vi "Dashboard Main.vi"() -> ()   [LabVIEW 2016]
uses:
  <vilib>/Utility/miscctls.llb/LVRowAndColumnTypeDef.ctl
  <vilib>/event_ctls.llb/eventvkey.ctl
  <vilib>/Rock Robotics/Network Tables/NT Read Numeric Array.vi
  <vilib>/Rock Robotics/Network Tables/NT Read Boolean.vi
  <vilib>/Rock Robotics/WPI/Dashboard/WPI_DashboardLogging Global.vi
panel:
  in  "Camera Settings Right":T1={"Frame Rate"=30, "Compression"=30, "Size"=1, "DB Camera Config"=FALSE} {"Frame Rate" scale=1.0..30.0; "Compression" scale=100.0..-1.0; "Size" items=["640x480", "320x240", "160x120"]}
  in  "Camera Name Right":string(combo)="No Camera Selection"
  out "Camera Info":cluster{"Mbps LED":bool, "Mbps":dbl, "fps":dbl} {"fps" format="%#.1g"; "Mbps" format="%#.1g"}
  in  "Camera Settings":T1={"Frame Rate"=30, "Compression"=30, "Size"=1, "DB Camera Config"=FALSE} {"Frame Rate" scale=1.0..30.0; "Compression" scale=100.0..-1.0; "Size" items=["640x480", "320x240", "160x120"]}
  in  "TCP":refnum<k5>
  in  "Rec Mode":enum32{"Stop", "Record", "Playback"}(radio)
  out "Robot IP":string
  out "Image Message":string="Timeout in Camera Communications"
  in  "Dashboard Tab":T2(tab)
  out "Waveform Chart":dbl[][](graph)
  out "Good to Shoot?":bool
  out "NT Connection":bool
  out "MotorChart R":cluster{"Numeric":dbl, "Numeric":dbl}(graph)
  out "MotorChart L":cluster{"Numeric":dbl, "Numeric":dbl}(graph)
  out "MotorSliders R":cluster{"MotorSlide1":dbl, "MotorSlide2":dbl} {"MotorSlide2" scale=-1.0..1.0 scale format="%#_2e"; "MotorSlide1" scale=-1.0..1.0 scale format="%#_2e"}
  out "MotorSliders L":cluster{"MotorSlide1":dbl, "MotorSlide2":dbl} {"MotorSlide2" scale=-1.0..1.0 scale format="%#_2e"; "MotorSlide1" scale=-1.0..1.0 scale format="%#_2e"}
  out "Gyro":dbl(knob) scale=0.0..360.0
  out "JS1 Z":dbl(slide) scale=-1.0..1.0 scale format="%#_2e"
  out "JS1 Graph":cluster{"X":dbl, "Y":dbl}[](graph)
  out "JS1 Buttons":T3
  out "JS2 Z":dbl(slide) scale=-1.0..1.0 scale format="%#_2e"
  out "JS2 Graph":cluster{"X":dbl, "Y":dbl}[](graph)
  out "JS2 Buttons":T3
  out "Mode":T4(ring)=enum."Auto Disabled"
  in  "Auto List":string(combo)="Select Autonomous ..."
  out "Camera Image Right":T5(plugin-control)
  in  "DB/String 9":string
  in  "DB/String 8":string
  in  "DB/String 7":string
  in  "DB/String 6":string
  in  "DB/String 5":string
  in  "DB/String 4":string
  in  "DB/String 3":string
  in  "DB/String 2":string
  in  "DB/String 1":string
  in  "DB/String 0":string
  in  "DB/Slider 0":dbl(slide) scale=0.0..5.0
  in  "DB/Slider 1":dbl(slide) scale=0.0..5.0
  in  "DB/Slider 2":dbl(slide) scale=0.0..5.0
  in  "DB/Slider 3":dbl(slide) scale=0.0..5.0
  out "DB/LED 3":bool
  out "DB/LED 2":bool
  out "DB/LED 1":bool
  out "DB/LED 0":bool
  in  "DB/Button 3":bool
  in  "DB/Button 2":bool
  in  "DB/Button 1":bool
  in  "DB/Button 0":bool caption="New Name"
  in  "Test Slider":dbl(slide) scale=0.0..100.0 scale format="%#_3g"
  in  "On/Off":bool caption="Solenoid"
  in  "Test Name":u16(ring) items=["Select the test to run..."]
  in  "Test Tree":string(tree)
  in  "Motor":cluster{"Value":dbl, "Enable":bool} {"Value" scale=-1.0..1.0 scale format="%#_3g"}
  out "Progress":T6 {"Test Progress" scale=0.0..100.0}
  in  "Rev/Fwd":cluster{"Forward":bool, "Reverse":bool}
  in  "Test Ring":u16(ring) items=["Monochrome", "Color"]
  out "Cmd Status":string
  in  "Execute Command":bool
  in  "Command Params":string[][](table)
  in  "Command Selection":i32(listbox)
  in  "CheckList":i32(listbox)
  out "Tree":string(tree)
  out "Camera Image":T5(plugin-control)
  out "Background":bool
  in  "Camera Name":string(combo)="No Camera Selection"
  # "HW"
  # "HW"
  # "Joysticks"
  # "Drive Motors"
  # "Front"
  # "Right"
  # "Left"
  # "Back"
  # "This tab is a great place for autonomous settings and robot-specific values.\nPlace controls and indicators inside this tab and match name to\nDashboard Variables on robot. You can also delete this comment."
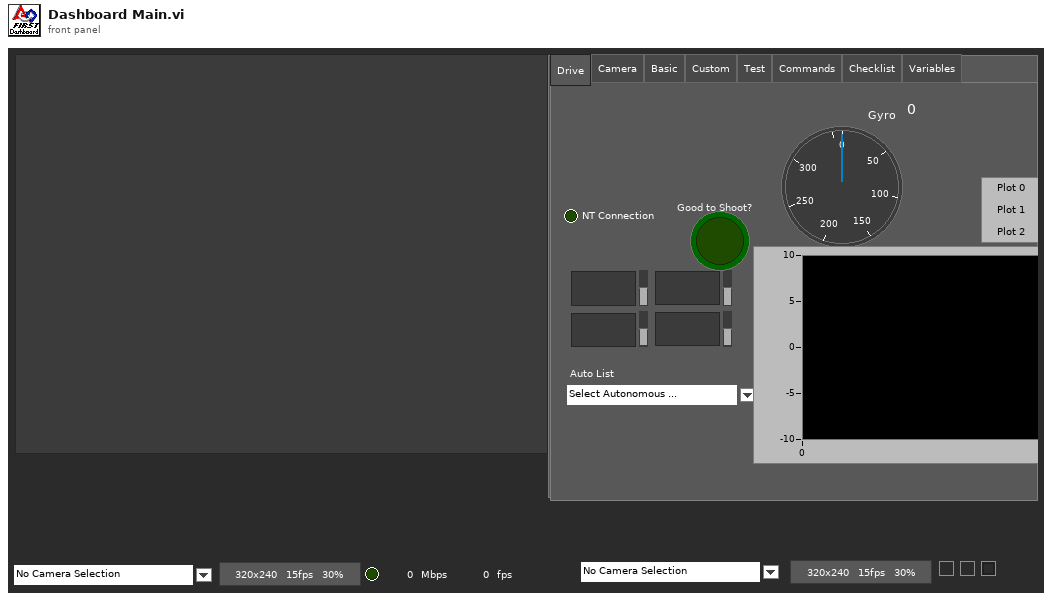
[diagram p1: front panel]
types:
  T1 = cluster{"Frame Rate":i32, "Compression":i32, "Size":u16, "DB Camera Config":bool}
  T2 = enum32{"Drive", "Camera", "Basic", "Custom", "Test", "Commands", "Checklist", "Variables"}
  T3 = cluster{bool, bool, bool, bool, bool, bool, bool, bool, bool, bool, bool, bool}
  T4 = enum8{"Tele-Op Disabled", "Tele-Op Enabled", "Auto Disabled", "Auto Enabled", "Test Disabled", "Test Enabled", "Disconnected", "No Code", "E-Stop"}
  T5 = typedef "IMAQ Image.ctl" = refnum<image>
  T6 = cluster{"Test Progress":u8, "Test Progress Text":string}
  T7 = typedef "Image Type" = u32
  T8 = cluster{"IDs":cluster{"RPC field ID":u16, "Unique ID":u16}, "String":string}
  T9 = enum32{"Drive", "Basic", "Custom", "Test", "Checklist", "Variables"}
  T10 = cluster{"Error Strings":string, "Disable Counts":cluster{u16, u16}, "Rail Faults":cluster{u16, u16, u16}, "Robot IP":string, "DB Mode":u8, "Event Info":cluster{"Name":string, "Type":u8, "Number":u16, "Replay":u8}}
  T11 = cluster{"Storage":cluster{"Disk Free":u64, "RAM Block":u32, "RAM free":u32}, "CPU Utilization":cluster{"CPU % ISR":sgl, "CPU % Time Crit":sgl, "CPU % Timed Str":sgl, "CPU % High":sgl, "CPU % Above":sgl, "CPU % Normal":sgl, "CPU % Low":sgl}, "CAN":cluster{"% Bus Utilization":sgl, "Bus Off Cnt":u32, "TX_FIFO Full Cnt":u32, "Receive Error Cnt":u8, "Transmit Error Cnt":u8}, "HID":cluster{"HID Outputs":u32, "Rumble Low":u16, "Rumble High":u16}[]}
  T12 = cluster{"Status bits":cluster{"Test Mode":bool, "Autonomous":bool, "Enabled":bool, "Code Start":bool, "Brownout":bool, "Reserved 2":bool, "Reserved 3":bool, "E-Stop":bool}, "Code Trace":cluster{"Disabled":bool, "TeleOp":bool, "Auto":bool, "Test":bool}, "Controller Type":enum16{"unknown", "cRIO", "roboRio"}, "Code?":enum16{"unknown", "noCode", "code"}, "Battery V":dbl}
  T13 = cluster{"Control Bits":cluster{"TestMode":bool, "Autonomous":bool, "Enabled":bool, "FMS Present":bool, bool, bool, bool, "E-Stop":bool}, "Team Station ":u8, "Countdown":sgl, "Joystick Values":cluster{"Axes":dbl[], "Buttons":bool[], "POVs":i16[]}[]}
  T14 = cluster{"Axes":dbl[], "Buttons":bool[], "POVs":i16[]}[]
  T15 = cluster{"Axes":dbl[], "Buttons":bool[], "POVs":i16[]}
  T16 = cluster{"Buttons[0]":bool, "Buttons[1]":bool, "Buttons[2]":bool, "Buttons[3]":bool, "Buttons[4]":bool, "Buttons[5]":bool, "Buttons[6]":bool, "Buttons[7]":bool, "Buttons[8]":bool, "Buttons[9]":bool, "Buttons[10]":bool, "Buttons[11]":bool}
  T17 = cluster{"Camera Image":refnum<vi>, "Dashboard Tab":refnum<vi>, "Background":refnum<vi>, "Rec Mode":refnum<vi>, "Test Slider":refnum<vi>, "On/Off ":refnum<vi>, "Test Ring":refnum<vi>, "Rev/Fwd":refnum<vi>, "Test Name":refnum<vi>, "Motor":refnum<vi>, "Progress":refnum<vi>, "CheckList":refnum<vi>, "Tree":refnum<vi>, "Test Tree":refnum<vi>, "Command Params":refnum<vi>, "Command Selection":refnum<vi>, "Execute Command":refnum<vi>, "Cmd Status":refnum<vi>, "Camera Settings":refnum<vi>, "Camera Name":refnum<vi>, "Camera Info":refnum<vi>, "Camera Settings Right":refnum<vi>, "Camera Name Right":refnum<vi>, "Camera Image Right":refnum<vi>}
  T18 = cluster{"Operation":enum16{"Update", "Clear"}, "Color Box":u32}[]
  T19 = typedef "eventvkey.ctl" = enum16{"ASCII", "Enter", "Return", "Shift", "Ctrl", "Alt", "Cmd", "Opt", "Caps", "NumLock", "Clear", "Break", "Up", "Down", "Left", "Right", "Insert", "Delete", "Home", "End", "PageUp", "PageDown", "Escape", "Help", "Pause", "ScrollLock", "F1", "F2", "F3", "F4", "F5", "F6", "F7", "F8", "F9", "F10", "F11", "F12", "F13", "F14", "F15", "F16", "F17", "F18", "F19", "F20", "F21", "F22", "F23", "F24", "Play", "VolumeUp", "VolumeDown", "Mute", "Two Byte Char"}
  T20 = cluster{"Image Size":bool, "Image Type":bool, "Pixel Value":bool, "ROI Information":bool, "Zoom Factor":bool}
  T21 = cluster{"Operation":enum16{"Update", "Clear"}, "Color Box":u32}
  T22 = typedef "LVRowAndColumnTypeDef.ctl" = cluster{"Row":i32, "Column":i32}
  T23 = cluster{"Shift":bool, "Ctrl":bool, "Alt":bool, "Cmd":bool, "Opt":bool}
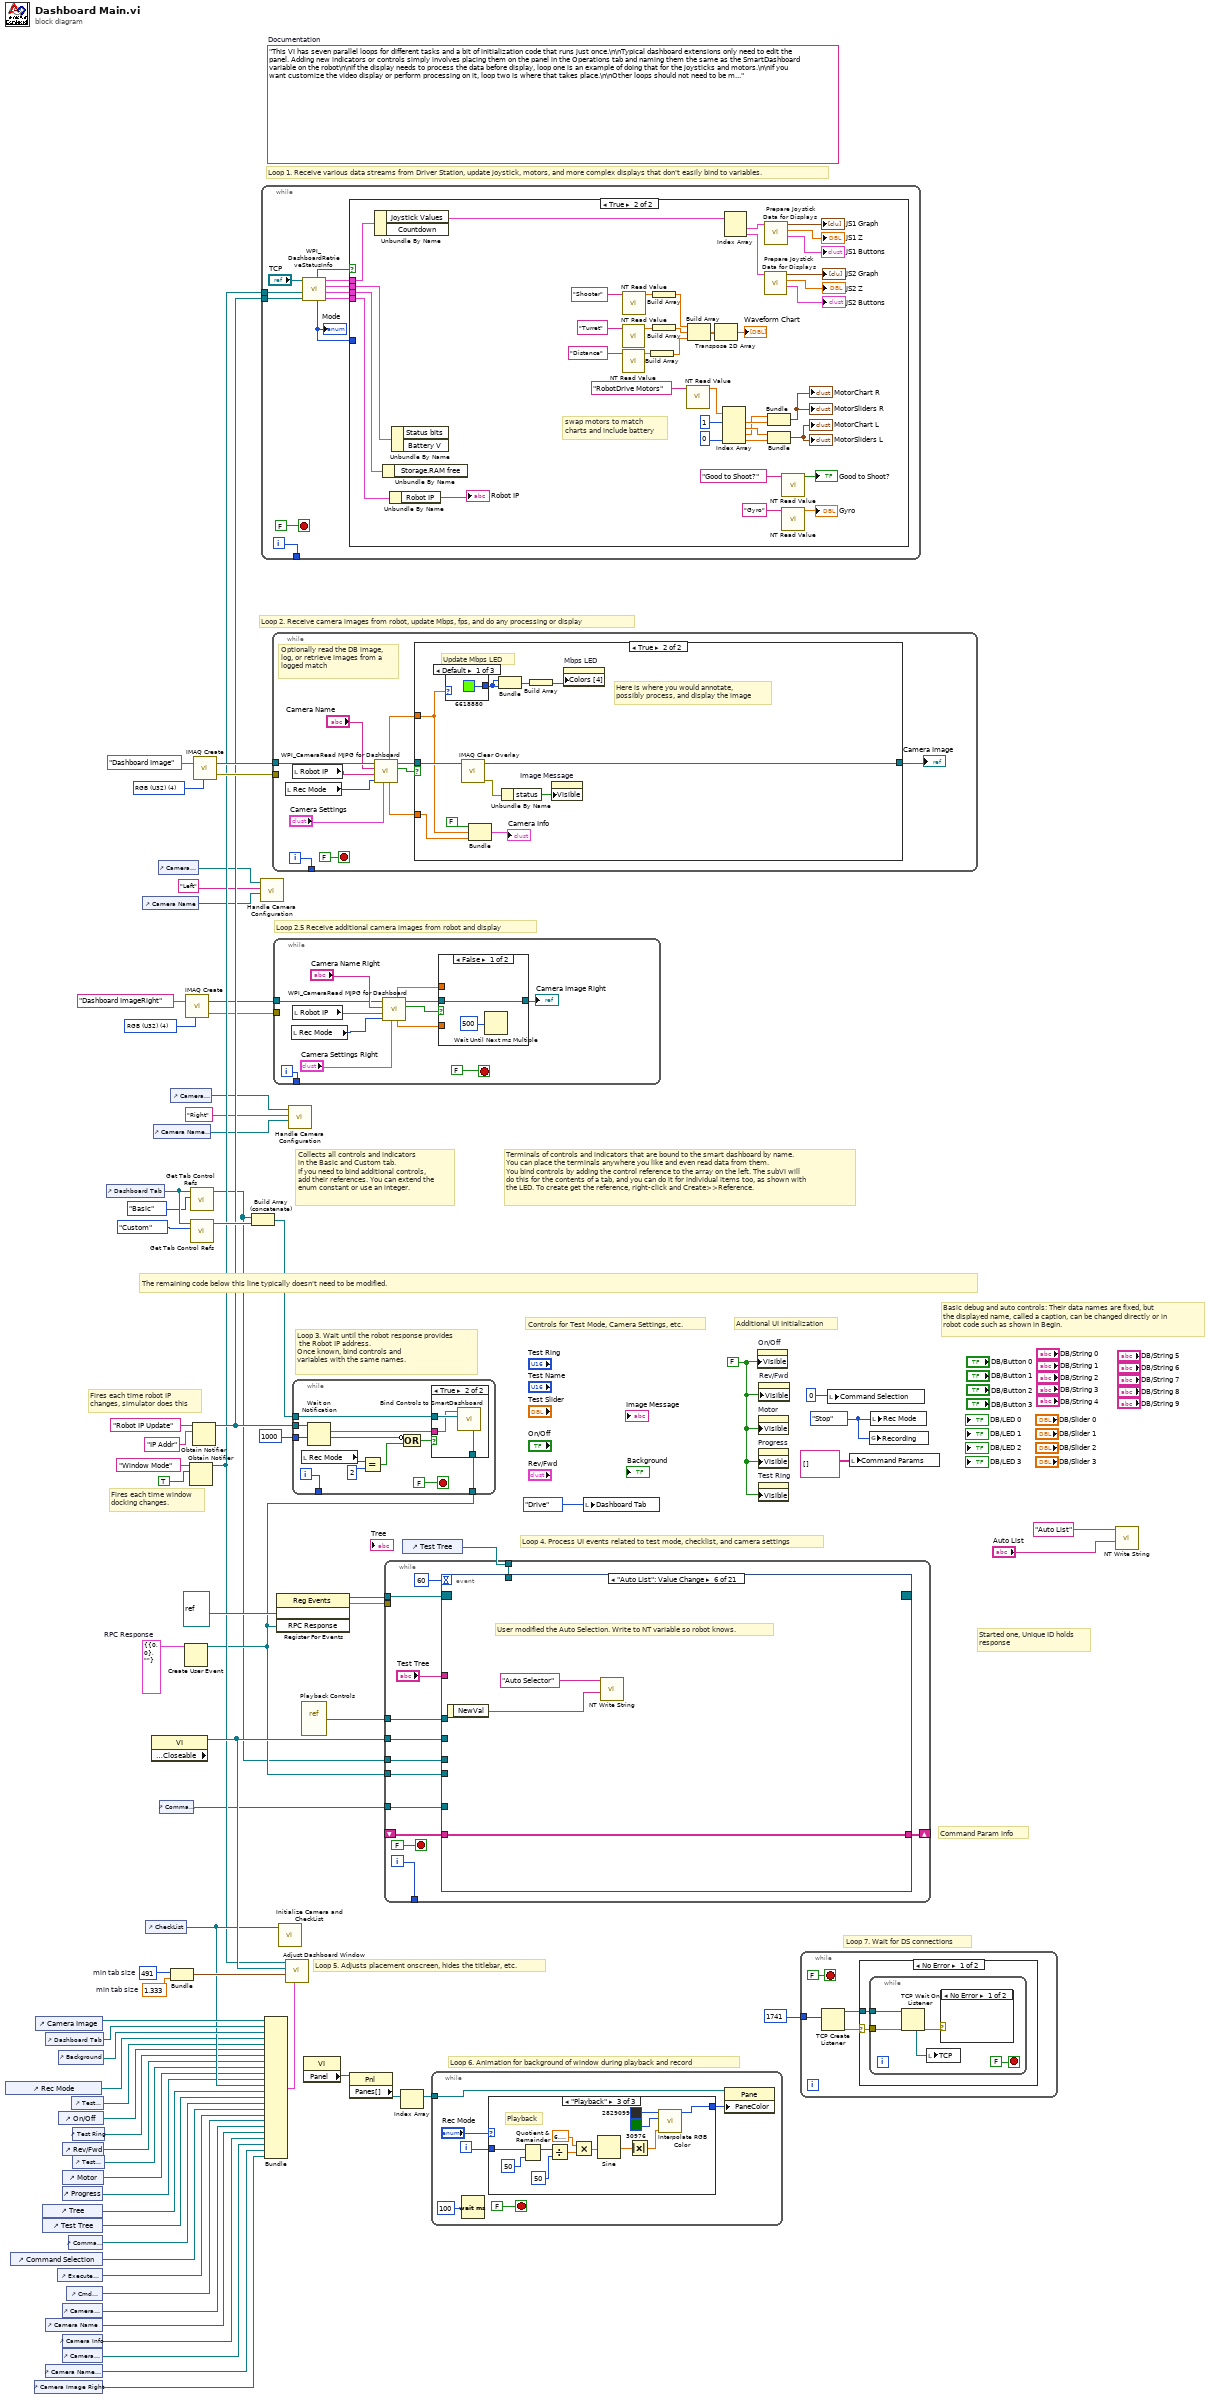
[diagram p0: block diagram]
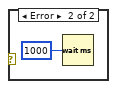
[diagram p3: hidden frame]
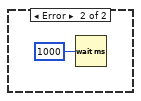
[diagram p4: hidden frame]
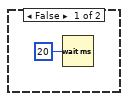
[diagram p5: hidden frame]
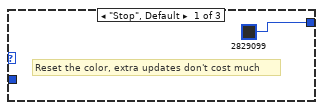
[diagram p6: hidden frame]
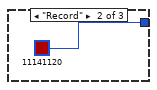
[diagram p7: hidden frame]
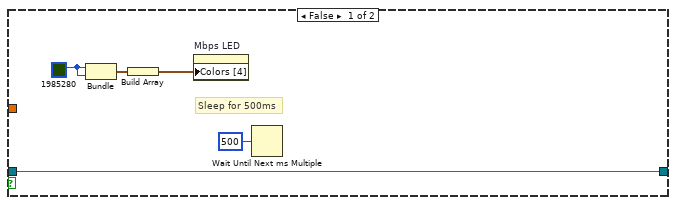
[diagram p9: hidden frame]
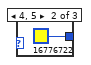
[diagram p10: hidden frame]
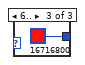
[diagram p11: hidden frame]
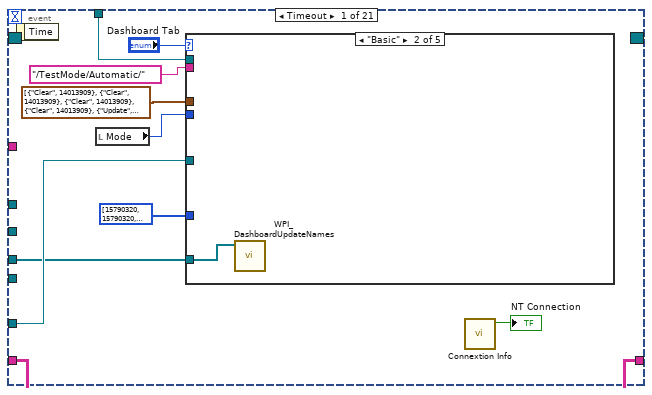
[diagram p12: hidden frame]
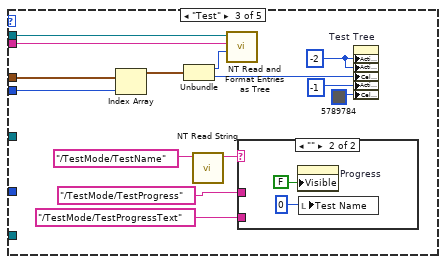
[diagram p14: hidden frame]
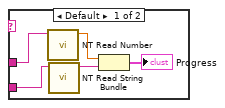
[diagram p15: hidden frame]
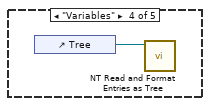
[diagram p16: hidden frame]
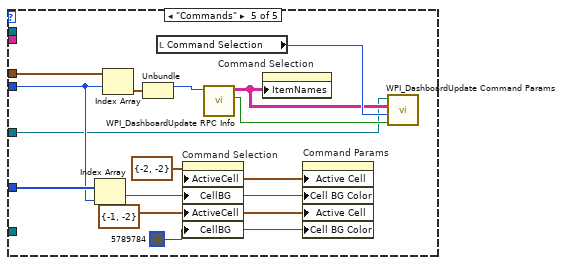
[diagram p17: hidden frame]
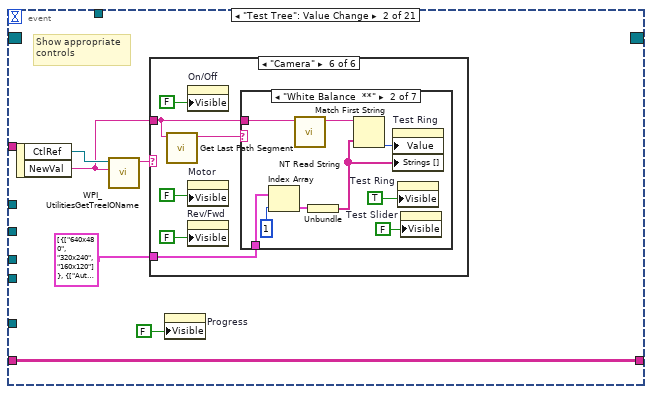
[diagram p18: hidden frame]
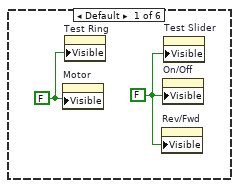
[diagram p19: hidden frame]
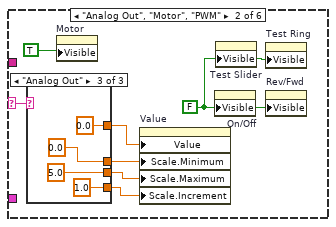
[diagram p20: hidden frame]
diagram:
  w12 = T7 4 items=["Grayscale (U8)", "Grayscale (I16)", "Grayscale (SGL)", "Complex (CSG)", "RGB (U32)", "HSL (U32)", "RGB (U64)"] ("Image Type")
  w26 = T8 {"IDs"={"RPC field ID"=0, "Unique ID"=0}, "String"=""}  # RPC Response
  w51 = 491  # min tab size
  w50 = 1.333  # min tab size
  w58 = enum32{"Stop", "Record", "Playback"}."Stop" ("Rec Mode")
  w33 = FALSE ("Visible")
  (unwired) "This VI has seven parallel loops for different tasks and a bit of initialization code that runs just once.\n\nTypical dashboard extensions only need to edit the panel. Adding new indicators or controls simply involves placing them on the panel in the Operations tab and naming them the same as the SmartDashboard variable on the robot\n\nIf the display needs to process the data before display, loop one is an example of doing that for the joysticks and motors.\n\nIf you want customize the video display or perform processing on it, loop two is where that takes place.\n\nOther loops should not need to be modified. They are pretty standard, and document the task they perform."  # Documentation
  w75 = T7 4 items=["Grayscale (U8)", "Grayscale (I16)", "Grayscale (SGL)", "Complex (CSG)", "RGB (U32)", "HSL (U32)", "RGB (U64)"] ("Image Type")
  # "Loop 2.5 Receive additional camera images from robot and display"
  # "Command Param Info"
  # "Started one, Unique ID holds\nresponse"
  # "Loop 7. Wait for DS connections"
  # "Basic debug and auto controls: Their data names are fixed, but\nthe displayed name, called a caption, can be changed directly or in\nrobot code such as shown in Begin."
  # "Controls for Test Mode, Camera Settings, etc."
  # "Additional UI Initialization"
  # "Loop 6. Animation for background of window during playback and record"
  # "Fires each time robot IP\nchanges, simulator does this"
  # "Fires each time window\ndocking changes."
  # "Collects all controls and indicators\nin the Basic and Custom tab.\nIf you need to bind additional controls,\nadd their references. You can extend the\nenum constant or use an integer."
  # "The remaining code below this line typically doesn't need to be modified."
  # "Loop 4. Process UI events related to test mode, checklist, and camera settings"
  # "Terminals of controls and indicators that are bound to the smart dashboard by name.\nYou can place the terminals anywhere you like and even read data from them.\nYou bind controls by adding the control reference to the array on the left. The subVI will\ndo this for the contents of a tab, and you can do it for individual items too, as shown with\nthe LED. To create get the reference, right-click and Create>>Reference."
  # "Loop 3. Wait until the robot response provides\n the Robot IP address.\nOnce known, bind controls and\nvariables with the same names."
  # "Loop 5. Adjusts placement onscreen, hides the titlebar, etc."
  # "Loop 1. Receive various data streams from Driver Station, update joystick, motors, and more complex displays that don't easily bind to variables."
  # "Loop 2. Receive camera images from robot, update Mbps, fps, and do any processing or display"
  n1 = control-ref of="Rec Mode"() -> (w39:refnum<vi>)
  n2 = control-ref of="Command Selection"() -> (w25:refnum<vi>)
  n3 = control-ref of="Camera Image Right"() -> (w3:refnum<vi>)
  n4 = control-ref of="Camera Image"() -> (w53:refnum<vi>)
  n5 = control-ref of="Tree"() -> (w43:refnum<vi>)
  n6 = control-ref of="Test Tree"() -> (w42:refnum<vi>)
  n7 = control-ref of="Dashboard Tab"() -> (w52:refnum<vi>)
  n8 = control-ref of="Camera Name"() -> (w16:refnum<vi>)
  n9 = control-ref of="Camera Name Right"() -> (w4:refnum<vi>)
  n10 = control-ref of="Execute Command"() -> (w27:refnum<vi>)
  n11 = control-ref of="Background"() -> (w48:refnum<vi>)
  n12 = control-ref of="On/Off"() -> (w37:refnum<vi>)
  n13 = control-ref of="Progress"() -> (w34:refnum<vi>)
  n14 = control-ref of="Camera Settings"() -> (w17:refnum<vi>)
  n15 = control-ref of="Camera Info"() -> (w15:refnum<vi>)
  n16 = control-ref of="Camera Settings Right"() -> (w5:refnum<vi>)
  n17 = control-ref of="Rev/Fwd"() -> (w35:refnum<vi>)
  n18 = control-ref of="Motor"() -> (w40:refnum<vi>)
  n19 = control-ref of="Cmd Status"() -> (w21:refnum<vi>)
  n20 = control-ref of="Command Params"() -> (w28:refnum<vi>)
  n21 = control-ref of="Test Slider"() -> (w38:refnum<vi>)
  n22 = control-ref of="Test Ring"() -> (w36:refnum<vi>)
  n23 = control-ref of="Test Name"() -> (w41:refnum<vi>)
  n24 = control-ref of="Dashboard Tab"() -> (w56:refnum<vi>)
  n25 = control-ref of="Camera Name"() -> (w18:refnum<vi>)
  n26 = control-ref of="CheckList"() -> (w44:refnum<vi>)
  n27 = property class="VI" props=["Front Panel.Closeable"]() -> (reference out=w57:refnum<vi>)  [unwired: 2 in, 2 out]
  n28 = control-ref of="Camera Name Right"() -> (w8:refnum<vi>)
  n29 = control-ref of="Camera Settings"() -> (w19:refnum<vi>)
  n30 = control-ref of="Command Params"() -> (w20:refnum<vi>)
  n31 = control-ref of="Camera Settings Right"() -> (w9:refnum<vi>)
  n32 = Bundle("min tab size"=w51, "min tab size"=w50) -> (w49:cluster{"min tab size":i32, "min tab size":dbl})  [unwired: 1 in]
  n33 = Create User Event(user event datatype=w26) -> (user event=w22:refnum<user-event>)  [unwired: 1 in, 1 out]
  n34 = call "IMAQ Create"("Image Name"="Dashboard ImageRight", "Image Type"=w12) -> ("New Image"=w11:T5, "error out"=w10:errorcluster)  [unwired: 2 in, 1 out]
  n35 = Obtain Notifier(name (unnamed)="Window Mode", notification data type=TRUE) -> (notifier out=w31:refnum<notifier>)  [unwired: 2 in, 2 out]
  n36 = call <vilib>:"Get Tab Control Refs.vi"("Page Index"=T9."Basic" ("Dashboard Tab"), "TabControl in"=w56) -> ("ControlsOnPage"=w14:refnum<vi>[])  [unwired: 9 in]
  n37 = call <vilib>:"Get Tab Control Refs.vi"("Page Index"=T9."Custom" ("Dashboard Tab"), "TabControl in"=w56) -> ("ControlsOnPage"=w55:refnum<vi>[])  [unwired: 9 in]
  n38 = Obtain Notifier(name (unnamed)="Robot IP Update", notification data type="IP Addr" ("name (unnamed)")) -> (notifier out=w32:refnum<notifier>)  [unwired: 2 in, 2 out]
  n39 = call "IMAQ Create"("Image Name"="Dashboard Image", "Image Type"=w75) -> ("New Image"=w73:T5, "error out"=w72:errorcluster)  [unwired: 2 in, 1 out]
  n40 = Build Array (concatenate)(w14, w55) -> (w54:refnum<vi>[])
  n41 = call "Handle Camera Configuration.vi"("CameraNameRef"=w18, "Camera File Name"="Left", "ClusterRef"=w19) -> ()  [unwired: 9 in]
  n42 = while {
    tunnel: [w85] -> _
    tunnel: w32 -> [w79]
    tunnel: w31 -> [w76]
    i -> [w85]
    stop <- FALSE stop-if-true
    n43 = call <vilib>:"WPI_DashboardRetrieveStatusInfo.vi"("Binding Refnum"=w79, "Window Mode Notifier"=w76, "TCP Cnx"="TCP") -> ("Power and Errors"=w80:T10, "Robot Metrics"=w83:T11, "Status Info"=w84:T12, "Control Info"=w81:T13, "Robot Mode"=w78:T4, "Process?"=w82:bool)  [unwired: 3 in]
    "Mode" <- w78
    n44 = case shown="True" w82 {
      tunnel: w84 -> [_ w126]
      tunnel: w83 -> [_ w125]
      tunnel: w81 -> [_ w124]
      tunnel: w80 -> [_ w123]
      tunnel: w78 -> [_ _]
      frame False {
        n45 = Wait (ms)(milliseconds to wait=u32 20) -> ()  [unwired: 1 out]
      }
      frame True {
        # "swap motors to match\ncharts and include battery"
        n46 = Unbundle By Name(w124) -> ("Joystick Values"=w114:T14)  [unwired: 1 out]
        n47 = Unbundle By Name(w125) -> ()  [unwired: 1 out]
        n48 = Unbundle By Name(w123) -> ("Robot IP"=→"Robot IP":string)
        n49 = Unbundle By Name(w126) -> ()  [unwired: 2 out]
        n50 = call-poly <vilib>:"NT Read Value.vi"("Name"="Turret") -> ("Numeric"=w94:dbl)  [unwired: 9 in, 1 out]
        n51 = call-poly <vilib>:"NT Read Value.vi"("Name"="Distance") -> ("Numeric"=w93:dbl)  [unwired: 9 in, 1 out]
        n52 = call-poly <vilib>:"NT Read Value.vi"("Name"="Shooter") -> ("Numeric"=w95:dbl)  [unwired: 9 in, 1 out]
        n53 = Build Array(w93) -> (w90:dbl[])
        n54 = Build Array(w95) -> (w92:dbl[])
        n55 = Build Array(w94) -> (w91:dbl[])
        n56 = call-poly <vilib>:"NT Read Value.vi"("Name"="RobotDrive Motors") -> ("Numeric Array"=w104:dbl[])  [unwired: 9 in, 1 out]
        n57 = Build Array(w92, w91, w90) -> (w89:dbl[][])
        n58 = Transpose 2D Array(2D array=w89) -> (transposed array=→"Waveform Chart":dbl[][])
        n59 = Index Array(array=w104, index #1=1, index #4=0) -> (element #1=w118:dbl, element #2=w119:dbl, element #3=w117:dbl, element #4=w122:dbl)  [unwired: 2 in]
        n60 = Index Array(array=w114) -> (element #1=w113:T15, element #2=w109:T15)  [unwired: 2 in]
        n61 = call "Prepare Joystick Data for Displays.vi"("Joystick Values"=w109) -> ("Buttons"=→"JS2 Buttons":T16, "Z Axis"=→"JS2 Z":dbl, "Cartesian Data"=→"JS2 Graph":cluster{"X axis":dbl, "X axis":dbl}[])  [unwired: 8 in]
        n62 = call "Prepare Joystick Data for Displays.vi"("Joystick Values"=w113) -> ("Buttons"=→"JS1 Buttons":T16, "Z Axis"=→"JS1 Z":dbl, "Cartesian Data"=→"JS1 Graph":cluster{"X axis":dbl, "X axis":dbl}[])  [unwired: 8 in]
        n63 = Bundle("Numeric"=w117, "Numeric"=w118) -> (→"MotorChart R" →"MotorSliders R":cluster{"Numeric":dbl, "Numeric":dbl})  [unwired: 1 in]
        n64 = Bundle("Numeric"=w119, "Numeric"=w122) -> (→"MotorChart L" →"MotorSliders L":cluster{"Numeric":dbl, "Numeric":dbl})  [unwired: 1 in]
        n65 = call-poly <vilib>:"NT Read Value.vi"("Name"="Good to Shoot?") -> ("Boolean"=→"Good to Shoot?":bool)  [unwired: 9 in, 1 out]
        n66 = call-poly <vilib>:"NT Read Value.vi"("Name"="Gyro") -> ("Numeric"=→"Gyro":dbl)  [unwired: 9 in, 1 out]
      }
    }
  }
  n67 = Bundle("Camera Image"=w53, "Dashboard Tab"=w52, "Background"=w48, "Rec Mode"=w39, "Test Slider"=w38, "On/Off"=w37, "Test Ring"=w36, "Rev/Fwd"=w35, "Test Name"=w41, "Motor"=w40, "Progress"=w34, "CheckList"=w44, "Tree"=w43, "Test Tree"=w42, "Command Params"=w28, "Command Selection"=w25, "Execute Command"=w27, "Cmd Status"=w21, "Camera Settings"=w17, "Camera Name"=w16, "Camera Info"=w15, "Camera Settings Right"=w5, "Camera Name Right"=w4, "Camera Image Right"=w3) -> (w45:T17)  [unwired: 1 in]
  n68 = while {
    tunnel: w73 -> [w136]
    tunnel: w72 -> [_]
    tunnel: [w137] -> _
    i -> [w137]
    stop <- FALSE stop-if-true
    # "Optionally read the DB image,\nlog, or retrieve images from a\nlogged match"
    n69 = local read "Rec Mode"() -> (w132:enum32{"Stop", "Record", "Playback"})
    n70 = local read "Robot IP"() -> (w131:string)
    n71 = call <vilib>:"WPI_CameraRead MJPG for Dashboard.vi"("Camera Settings"="Camera Settings", "Rec Mode"=w132, "Robot IP"=w131, "Camera Name"="Camera Name", "Refnum in"=w136) -> ("Active"=w134:bool, "Refnum out"=w135:T5, "FPS"=w133:dbl, "Bandwidth (Mbps)"=w130:dbl)  [unwired: 3 in]
    n72 = case shown="True" w134 {
      tunnel: w135 -> [w139 w150]
      tunnel: w130 -> [_ w147]
      tunnel: w133 -> [_ w148]
      tunnel: [w139 w144] -> w127
      frame False {
        w141 = u32 1985280 ("Color Box")
        # "Sleep for 500ms"
        n73 = Bundle("Color Box"=w141, "Color Box"=w141) -> (w142:cluster{"Color Box":u32, "Color Box":u32})  [unwired: 1 out]
        n74 = Build Array(w142) -> (w140:cluster{"Color Box":u32, "Color Box":u32}[])
        n75 = property on="Mbps LED" class="Bool (strict)"("Colors [4]"=w140) -> ()  [unwired: 2 in, 2 out]
        n76 = Wait Until Next ms Multiple(millisecond multiple=u32 500) -> ()  [unwired: 1 out]
      }
      frame True {
        # "Here is where you would annotate,\npossibly process, and display the image"
        # "Update Mbps LED"
        n77 = case shown="Default" w147 {
          tunnel: [u32 6618880 ("Color Box") u32 16776722 ("Color Box") u32 16716800 ("Color Box")] -> w151
          frame Default {
          }
          frame 4, 5 {
          }
          frame 6.. {
          }
        }
        n78 = call "IMAQ Clear Overlay"("Image"=w150) -> ("error out"=w153:errorcluster, "Image Out"=w144:T5)  [unwired: 2 in, 7 out]
        n79 = Bundle(FALSE, "Bandwidth (Mbps)"=w147, "FPS"=w148) -> (→"Camera Info":cluster{bool, "Bandwidth (Mbps)":dbl, "FPS":dbl})  [unwired: 1 in]
        n80 = Bundle("Color Box"=w151, "Color Box"=w151) -> (w152:cluster{"Color Box":u32, "Color Box":u32})  [unwired: 1 out]
        n81 = Unbundle By Name(w153) -> ("status"=w154:bool)
        n82 = Build Array(w152) -> (w149:cluster{"Color Box":u32, "Color Box":u32}[])
        n83 = property on="Image Message" class="Str"("Visible"=w154) -> ()  [unwired: 2 in, 2 out]
        n84 = property on="Mbps LED" class="Bool (strict)"("Colors [4]"=w149) -> ()  [unwired: 2 in, 2 out]
      }
    }
    "Camera Image" <- w127
  }
  n85 = while {
    tunnel: w11 -> [w168]
    tunnel: w10 -> [_]
    tunnel: [w162] -> _
    i -> [w162]
    stop <- FALSE stop-if-true
    n86 = local read "Rec Mode"() -> (w166:enum32{"Stop", "Record", "Playback"})
    n87 = local read "Robot IP"() -> (w167:string)
    n88 = call <vilib>:"WPI_CameraRead MJPG for Dashboard.vi"("Camera Settings"="Camera Settings Right", "Rec Mode"=w166, "Robot IP"=w167, "Camera Name"="Camera Name Right", "Refnum in"=w168) -> ("Active"=w161:bool, "Refnum out"=w164:T5, "FPS"=w159:dbl, "Bandwidth (Mbps)"=w160:dbl)  [unwired: 3 in]
    n89 = case shown="False" w161 {
      tunnel: w164 -> [w170 w172]
      tunnel: w160 -> [_ _]
      tunnel: w159 -> [_ _]
      tunnel: [w170 w172] -> w158
      frame False {
        n90 = Wait Until Next ms Multiple(millisecond multiple=u32 500) -> ()  [unwired: 1 out]
      }
      frame True {
      }
    }
    "Camera Image Right" <- w158
  }
  n91 = register-events(refnum<vi> refnum, w22) -> (reference out=w62:refnum<event-registration>, error out=w61:errorcluster)  [unwired: 2 in]
  n92 = call "Initialize Camera and CheckList.vi"("ListBox in"=w44) -> ()  [unwired: 11 in]
  n93 = call "Adjust Dashboard Window.vi"("Sizing Refnums"=w45, "Size Constraints"=w49, "VI"=w57, "WIn Mode"=w31) -> ()  [unwired: 8 in]
  n94 = call "Handle Camera Configuration.vi"("CameraNameRef"=w8, "Camera File Name"="Right", "ClusterRef"=w9) -> ()  [unwired: 9 in]
  n95 = while {
    tunnel: w54 -> [w184]
    tunnel: w32 -> [w182]
    tunnel: [w180] -> _
    tunnel: u32 1000 ("milliseconds to wait") -> [w179]
    tunnel: w22 -> [w173]
    i -> [w180]
    stop <- FALSE stop-if-true
    n96 = local read "Rec Mode"() -> (w175:enum32{"Stop", "Record", "Playback"})
    n97 = Wait on Notification(notifier=w182, timeout in ms (-1)=w179) -> (notification=w181:string, timed out?=w177:bool)  [unwired: 2 in, 2 out]
    n98 = Equal?(x=w175, y=u16 2 ("Rec Mode")) -> (x = y?=w176:bool)
    n99 = Compound Arithmetic op=OR(invert w177, w176) -> (w178:bool)
    n100 = case shown="True" w178 {
      tunnel: w184 -> [_ w187]
      tunnel: w181 -> [_ w186]
      tunnel: w173 -> [_ w185]
      frame False {
      }
      frame True {
        n101 = call <vilib>:"Bind Controls to SmartDashboard.vi"("RPC ref"=w185, "Bound Control Refs"=w187, "Server IP Address"=w186) -> ()  [unwired: 9 in]
      }
    }
  }
  n102 = vi-ref "Playback Controls.vi"() -> (w63:refnum<vi>)
  n103 = property class="VI"() -> ("Panel"=w65:refnum<vi>)  [unwired: 2 in, 2 out]
  n104 = property class="Pnl"(reference=w65) -> ("Panes[]"=w66:refnum<vi>[])  [unwired: 1 in, 2 out]
  n105 = Index Array(array=w66) -> (element=w64:refnum<vi>)  [unwired: 1 in]
  n106 = control-ref of="Test Tree"() -> (w67:refnum<vi>)
  n107 = while {
    tunnel: [w197] -> _
    tunnel: w67 -> [w196]
    tunnel: w63 -> [w195]
    tunnel: w62 -> [w194]
    tunnel: w61 -> [_]
    tunnel: w57 -> [w193]
    tunnel: w22 -> [w192]
    tunnel: w20 -> [w191]
    shift-right: [w190] -> _
    shift-left: _ -> [w189]
    tunnel: w14 -> [w188]
    i -> [w197]
    stop <- FALSE stop-if-true
    n108 = event shown="[5] \"Auto List\": Value Change" {
      selector: w194 -> [_ _ _ _ _ _ _ _ _ _ _ _ _ _ _ _ _ _ _ _ _]
      dyn-events: [_ _ _ _ _ _ _ _ _ _ _ _ _ _ _ _ w453 _ _ _ _] -> _
      timeout: u32 60 ("milliseconds to wait") -> [_ _ _ _ _ _ _ _ _ _ _ _ _ _ _ _ _ _ _ _ _]
      tunnel: w196 -> [w209 _ _ _ _ _ _ _ _ _ _ _ _ _ _ _ _ _ _ _ _]
      tunnel: "Test Tree" -> [_ _ _ _ _ _ _ _ _ _ _ w420 w428 w430 w434 w442 _ _ _ _ _]
      tunnel: w195 -> [_ _ _ _ _ _ _ _ _ _ _ _ _ _ _ _ w455 _ w473 _ _]
      tunnel: w193 -> [_ _ _ _ _ _ _ _ _ _ _ _ _ _ _ _ w451 _ _ _ _]
      tunnel: w192 -> [_ _ _ _ _ _ _ _ _ _ _ _ _ _ _ _ w447 _ _ _ _]
      tunnel: w191 -> [w204 _ _ _ _ _ w371 _ _ _ _ _ _ _ _ _ _ _ _ _ _]
      tunnel: [w203 w248 w350 w355 w364 w368 w369 w378 w388 w395 w407 w419 w426 w429 w433 w441 w446 w468 w470 w474 w485] -> w190
      tunnel: w189 -> [w203 w248 w350 w355 w364 w368 w369 _ _ w395 w407 w419 w426 w429 w433 w441 w446 w468 w470 w474 w485]
      tunnel: w188 -> [w201 _ _ _ _ _ _ _ _ _ _ _ _ _ _ _ _ _ _ _ _]
      event Timeout {
        n109 = event-data() -> ()  [unwired: 1 in, 1 out]
        n110 = local read "Mode"() -> (w206:T4)
        n111 = case shown="\"Basic\"" "Dashboard Tab" {
          tunnel: w209 -> [_ _ w225 _ _]
          tunnel: "/TestMode/Automatic/" ("Name Pattern") -> [_ _ w224 _ _]
          tunnel: T18 [{"Operation"=enum."Clear", "Color Box"=14013909}, {"Operation"=enum."Clear", "Color Box"=14013909}, {"Operation"=enum."Clear", "Color Box"=14013909}, {"Operation"=enum."Clear", "Color Box"=14013909}, {"Operation"=enum."Update", "Color Box"=14013909}, {"Operation"=enum."Update", "Color Box"=16777215}, {"Operation"=enum."Clear", "Color Box"=14013909}, {"Operation"=enum."Clear", "Color Box"=14013909}, {"Operation"=enum."Clear", "Color Box"=14013909}] -> [_ _ w217 _ w241]
          tunnel: w206 -> [_ _ w216 _ w240]
          tunnel: u32[] [15790320, 15790320, 15790320, 15790320, 16777215, 16777215, 15790320, 15790320, 15790320] -> [_ _ _ _ w246]
          tunnel: w204 -> [_ _ _ _ w234]
          tunnel: w201 -> [_ w211 _ _ _]
          frame "Custom", Default {
          }
          frame "Basic" {
            n112 = call <vilib>:"WPI_DashboardUpdateNames.vi"("Controls on Tab"=w211) -> ()  [unwired: 11 in]
          }
          frame "Test" {
            w223 = -2 ("Active Item:Row Number")
            n113 = Index Array(array=w217, index=w216) -> (element=w218:T21)
            n114 = Unbundle(w218) -> ("Operation"=w219:enum16{"Update", "Clear"}, "Color Box"=w220:u32)
            n115 = call <vilib>:"NT Read String.vi"("Name"="/TestMode/TestName") -> ("String"=w214:string)  [unwired: 9 in, 1 out]
            n116 = call <vilib>:"NT Read and Format Entries as Tree.vi"("Operation"=w219, "Name Pattern"=w224, "Tree Refnum"=w225) -> ()  [unwired: 7 in, 2 out]
            n117 = case shown="\"\"" w214 {
              tunnel: "/TestMode/TestProgress" ("Name") -> [w227 _]
              tunnel: "/TestMode/TestProgressText" ("Name") -> [w226 _]
              frame Default {
                n118 = call <vilib>:"NT Read Number.vi"("Name"=w227) -> ("Numeric"=w228:dbl)  [unwired: 9 in, 1 out]
                n119 = call <vilib>:"NT Read String.vi"("Name"=w226) -> ("String"=w229:string)  [unwired: 9 in, 1 out]
                n120 = Bundle("Numeric"=w228, "String"=w229) -> (→"Progress":cluster{"Numeric":dbl, "String":string})  [unwired: 1 in]
              }
              frame "" {
                n121 = property on="Progress" class="Clust (strict)"("Visible"=FALSE) -> ()  [unwired: 2 in, 2 out]
                n122 = local write "Test Name"(u16 0) -> ()
              }
            }
            n123 = property on="Test Tree" class="Tree (strict)"("Active Item Row Number"=w223, "ActiveColNum"=w223, "CellBG"=w220, "Active Item Row Number"=-1 ("Active Item:Row Number"), "CellBG"=u32 5789784 ("Color Box")) -> ()  [unwired: 2 in, 2 out]
          }
          frame "Variables" {
            n124 = control-ref of="Tree"() -> (w233:refnum<vi>)
            n125 = call <vilib>:"NT Read and Format Entries as Tree.vi"("Tree Refnum"=w233) -> ()  [unwired: 9 in, 2 out]
          }
          frame "Commands" {
            w242 = u32 5789784 ("Color Box")
            w243 = T22 {"Row"=-1, "Column"=-2} ("Active Cell:Active Cell")
            w245 = T22 {"Row"=-2, "Column"=-2} ("Active Cell:Active Cell")
            n126 = Index Array(array=w246, index=w240) -> (element=w244:u32)
            n127 = Index Array(array=w241, index=w240) -> (element=w239:T21)
            n128 = Unbundle(w239) -> ("Operation"=w238:enum16{"Update", "Clear"})  [unwired: 1 out]
            n129 = local read "Command Selection"() -> (w237:i32)
            n130 = property on="Command Selection" class="MCListbox (strict)"("ActiveCell"=w245, "CellBG"=w244, "ActiveCell"=w243, "CellBG"=w242) -> ()  [unwired: 2 in, 2 out]
            n131 = call <vilib>:"WPI_DashboardUpdate RPC Info.vi"("Operation"=w238) -> ("update"=w236:bool, "commands"=w235:string[][])  [unwired: 9 in]
            n132 = property on="Command Selection" class="MCListbox (strict)"("ItemNames"=w235) -> ()  [unwired: 2 in, 2 out]
            n133 = property on="Command Params" class="Tbl (strict)"("Active Cell"=w245, "Cell BG Color"=w244, "Active Cell"=w243, "Cell BG Color"=w242) -> ()  [unwired: 2 in, 2 out]
            n134 = call <vilib>:"WPI_DashboardUpdate Command Params.vi"("Update"=w236, "NewVal"=w237, "Commands"=w235, "Param Tbl"=w234) -> ()  [unwired: 7 in, 1 out]
          }
        }
        n135 = call <vilib>:"Connextion Info.vi"() -> ("Connected"=→"NT Connection":bool)  [unwired: 10 in, 1 out]
      }
      event "Test Tree": Value Change {
        # "Show appropriate\ncontrols"
        n136 = event-data() -> ("CtlRef"=w251:refnum<vi>, "NewVal"=w249:string)  [unwired: 1 in]
        n137 = call <vilib>:"WPI_UtilitiesGetTreeIOName.vi"("NewVal"=w249, "TreeControl in"=w251) -> ("I/O Name"=w252:string)  [unwired: 9 in]
        n138 = case shown="\"Camera\"" w252 {
          selector: w252 -> [_ w259 _ w281 w290 _]
          tunnel: w249 -> [_ _ w278 w280 _ w297]
          tunnel: cluster{string[]}[] [{["640x480", "320x240", "160x120"]}, {["Auto", "Fixed indoor", "Fixed outdoor 1", "Fixed outdoor 2", "Fixed fluorescent 1", "Fixed fluorescent 2", "Hold current"]}, {["Auto", "Flicker-free 50 Hz", "Flicker-free 60 Hz", "Hold current"]}, {["None", "Prioritize frame rate", "Prioritize image quality"]}, {["Monochrome", "Color"]}] -> [_ _ _ _ _ w296]
          frame Default {
            w254 = FALSE ("Visible")
            w253 = FALSE ("Visible")
            n139 = property on="Motor" class="Clust (strict)"("Visible"=w253) -> ()  [unwired: 2 in, 2 out]
            n140 = property on="Test Ring" class="Ring (strict)"("Visible"=w253) -> ()  [unwired: 2 in, 2 out]
            n141 = property on="Rev/Fwd" class="Clust (strict)"("Visible"=w254) -> ()  [unwired: 2 in, 2 out]
            n142 = property on="On/Off" class="Bool (strict)"("Visible"=w254) -> ()  [unwired: 2 in, 2 out]
            n143 = property on="Test Slider" class="Slide (strict)"("Visible"=w254) -> ()  [unwired: 2 in, 2 out]
          }
          frame "Analog Out", "Motor", "PWM" {
            w260 = FALSE ("Visible")
            n144 = case shown="\"Analog Out\"" w259 {
              tunnel: [1.0 ("Value") -1.0 ("Value") 0.0 ("Value")] -> w258
              tunnel: [255.0 ("Value") 1.0 ("Value") 5.0 ("Value")] -> w257
              tunnel: [128.0 ("Value") 0.0 ("Value") 0.0 ("Value")] -> w256
              tunnel: [64.0 ("Value") 0.5 ("Value") 1.0 ("Value")] -> w255
              frame "PWM" {
              }
              frame "Motor", Default {
              }
              frame "Analog Out" {
              }
            }
            n145 = property on="Motor" class="Clust (strict)"("Visible"=TRUE) -> ()  [unwired: 2 in, 2 out]
            n146 = property on="Value" class="Slide (strict)"("Value"=w256, "Scale.Minimum"=w258, "Scale.Maximum"=w257, "Scale.Increment"=w255) -> ()  [unwired: 2 in, 2 out]
            n147 = property on="On/Off" class="Bool (strict)"("Visible"=w260) -> ()  [unwired: 2 in, 2 out]
            n148 = property on="Test Slider" class="Slide (strict)"("Visible"=w260) -> ()  [unwired: 2 in, 2 out]
            n149 = property on="Test Ring" class="Ring (strict)"("Visible"=w260) -> ()  [unwired: 2 in, 2 out]
            n150 = property on="Rev/Fwd" class="Clust (strict)"("Visible"=w260) -> ()  [unwired: 2 in, 2 out]
          }
          frame "Servo" {
            w276 = FALSE ("Visible")
            n151 = call <vilib>:"NT Read Number.vi"("Name"=w278) -> ("Numeric"=w277:dbl)  [unwired: 9 in, 1 out]
            n152 = property on="Test Slider" class="Slide (strict)"("Visible"=TRUE, "Scale.Maximum"=170.0 ("Scale.Range:Maximum")) -> ()  [unwired: 2 in, 2 out]
            n153 = local write "Test Slider"(w277) -> ()
            n154 = property on="Motor" class="Clust (strict)"("Visible"=w276) -> ()  [unwired: 2 in, 2 out]
            n155 = property on="Rev/Fwd" class="Clust (strict)"("Visible"=w276) -> ()  [unwired: 2 in, 2 out]
            n156 = property on="On/Off" class="Bool (strict)"("Visible"=w276) -> ()  [unwired: 2 in, 2 out]
            n157 = property on="Test Ring" class="Ring (strict)"("Visible"=w276) -> ()  [unwired: 2 in, 2 out]
          }
          frame "Relay", "Solenoid" {
            w279 = FALSE ("Visible")
            n158 = property on="Motor" class="Clust (strict)"("Visible"=w279) -> ()  [unwired: 2 in, 2 out]
            n159 = property on="Test Slider" class="Slide (strict)"("Visible"=w279) -> ()  [unwired: 2 in, 2 out]
            n160 = Search and Replace String(input string=w280, search string="/Value  **", replace string="/Direction") -> (result string=w286:string)  [unwired: 5 in, 3 out]
            n161 = property on="Test Ring" class="Ring (strict)"("Visible"=w279) -> ()  [unwired: 2 in, 2 out]
            n162 = call <vilib>:"NT Read String.vi"("Name"=w286) -> ("String"=w284:string)  [unwired: 9 in, 1 out]
            n163 = Equal?(x="Both directions", y=w284) -> (x = y?=w282:bool)
            n164 = Not(x=w282) -> (.not. x?=w283:bool)
            n165 = property on="Rev/Fwd" class="Clust (strict)"("Visible"=w282) -> ()  [unwired: 2 in, 2 out]
            n166 = property on="On/Off" class="Bool (strict)"("Visible"=w283, "Caption.Text"=w281) -> ()  [unwired: 2 in, 2 out]
          }
          frame "Compressor", "Digital Out" {
            w289 = FALSE ("Visible")
            # "Get direction and finish"
            n167 = property on="Motor" class="Clust (strict)"("Visible"=w289) -> ()  [unwired: 2 in, 2 out]
            n168 = property on="Test Slider" class="Slide (strict)"("Visible"=w289) -> ()  [unwired: 2 in, 2 out]
            n169 = property on="Test Ring" class="Ring (strict)"("Visible"=w289) -> ()  [unwired: 2 in, 2 out]
            n170 = property on="On/Off" class="Bool (strict)"("Visible"=TRUE, "Caption.Text"=w290) -> ()  [unwired: 2 in, 2 out]
            n171 = property on="Rev/Fwd" class="Clust (strict)"("Visible"=FALSE) -> ()  [unwired: 2 in, 2 out]
          }
          frame "Camera" {
            n172 = call <vilib>:"Get Last Path Segment.vi"("String in"=w297) -> ("String out"=w298:string)  [unwired: 10 in]
            n173 = property on="On/Off" class="Bool (strict)"("Visible"=FALSE) -> ()  [unwired: 2 in, 2 out]
            n174 = property on="Motor" class="Clust (strict)"("Visible"=FALSE) -> ()  [unwired: 2 in, 2 out]
            n175 = property on="Rev/Fwd" class="Clust (strict)"("Visible"=FALSE) -> ()  [unwired: 2 in, 2 out]
            n176 = case shown="\"White Balance  **\"" w298 {
              tunnel: w297 -> [w304 w313 w322 w331 w340 _ w346]
              tunnel: w296 -> [w302 w310 w319 w328 w337 _ _]
              frame "Size  **" {
                n177 = Index Array(array=w302) -> (element=w301:cluster{string[]})  [unwired: 1 in]
                n178 = call <vilib>:"NT Read String.vi"("Name"=w304) -> ("String"=w303:string)  [unwired: 9 in, 1 out]
                n179 = Unbundle(w301) -> (w299:string[])
                n180 = Match First String(2:w299, 3:w303) -> (0:w300:i32)  [unwired: 1 out]
                n181 = property on="Test Ring" class="Ring (strict)"("Value"=w300, "Strings []"=w299) -> ()  [unwired: 2 in, 2 out]
                n182 = property on="Test Ring" class="Ring (strict)"("Visible"=TRUE) -> ()  [unwired: 2 in, 2 out]
                n183 = property on="Test Slider" class="Slide (strict)"("Visible"=FALSE) -> ()  [unwired: 2 in, 2 out]
              }
              frame "White Balance  **" {
                n184 = Index Array(array=w310, index=1) -> (element=w311:cluster{string[]})
                n185 = call <vilib>:"NT Read String.vi"("Name"=w313) -> ("String"=w312:string)  [unwired: 9 in, 1 out]
                n186 = Unbundle(w311) -> (w308:string[])
                n187 = Match First String(2:w308, 3:w312) -> (0:w307:i32)  [unwired: 1 out]
                n188 = property on="Test Ring" class="Ring (strict)"("Value"=w307, "Strings []"=w308) -> ()  [unwired: 2 in, 2 out]
                n189 = property on="Test Ring" class="Ring (strict)"("Visible"=TRUE) -> ()  [unwired: 2 in, 2 out]
                n190 = property on="Test Slider" class="Slide (strict)"("Visible"=FALSE) -> ()  [unwired: 2 in, 2 out]
              }
              frame "Exposure  **" {
                n191 = Index Array(array=w319, index=2) -> (element=w320:cluster{string[]})
                n192 = call <vilib>:"NT Read String.vi"("Name"=w322) -> ("String"=w321:string)  [unwired: 9 in, 1 out]
                n193 = Unbundle(w320) -> (w316:string[])
                n194 = Match First String(2:w316, 3:w321) -> (0:w317:i32)  [unwired: 1 out]
                n195 = property on="Test Ring" class="Ring (strict)"("Value"=w317, "Strings []"=w316) -> ()  [unwired: 2 in, 2 out]
                n196 = property on="Test Ring" class="Ring (strict)"("Visible"=TRUE) -> ()  [unwired: 2 in, 2 out]
                n197 = property on="Test Slider" class="Slide (strict)"("Visible"=FALSE) -> ()  [unwired: 2 in, 2 out]
              }
              frame "Exposure Priority  **" {
                n198 = Index Array(array=w328, index=3) -> (element=w329:cluster{string[]})
                n199 = call <vilib>:"NT Read String.vi"("Name"=w331) -> ("String"=w330:string)  [unwired: 9 in, 1 out]
                n200 = Unbundle(w329) -> (w325:string[])
                n201 = Match First String(2:w325, 3:w330) -> (0:w326:i32)  [unwired: 1 out]
                n202 = property on="Test Ring" class="Ring (strict)"("Value"=w326, "Strings []"=w325) -> ()  [unwired: 2 in, 2 out]
                n203 = property on="Test Ring" class="Ring (strict)"("Visible"=TRUE) -> ()  [unwired: 2 in, 2 out]
                n204 = property on="Test Slider" class="Slide (strict)"("Visible"=FALSE) -> ()  [unwired: 2 in, 2 out]
              }
              frame "Color Enable  **" {
                n205 = Index Array(array=w337, index=4) -> (element=w338:cluster{string[]})
                n206 = call <vilib>:"NT Read String.vi"("Name"=w340) -> ("String"=w339:string)  [unwired: 9 in, 1 out]
                n207 = Unbundle(w338) -> (w334:string[])
                n208 = Match First String(2:w334, 3:w339) -> (0:w335:i32)  [unwired: 1 out]
                n209 = property on="Test Ring" class="Ring (strict)"("Value"=w335, "Strings []"=w334) -> ()  [unwired: 2 in, 2 out]
                n210 = property on="Test Ring" class="Ring (strict)"("Visible"=TRUE) -> ()  [unwired: 2 in, 2 out]
                n211 = property on="Test Slider" class="Slide (strict)"("Visible"=FALSE) -> ()  [unwired: 2 in, 2 out]
              }
              frame Default {
                n212 = property on="Test Ring" class="Ring (strict)"("Visible"=FALSE) -> ()  [unwired: 2 in, 2 out]
                n213 = property on="Test Slider" class="Slide (strict)"("Visible"=FALSE) -> ()  [unwired: 2 in, 2 out]
              }
              frame "Brightness  **", "Color Level  **", "Compression  **", "FPS  **", "Sharpness  **" {
                n214 = call <vilib>:"NT Read Number.vi"("Name"=w346) -> ("Numeric"=w345:dbl)  [unwired: 9 in, 1 out]
                n215 = local write "Test Slider"(w345) -> ()
                n216 = property on="Test Slider" class="Slide (strict)"("Visible"=TRUE, "Scale.Maximum"=100.0 ("Scale.Range:Maximum")) -> ()  [unwired: 2 in, 2 out]
                n217 = property on="Test Ring" class="Ring (strict)"("Visible"=FALSE) -> ()  [unwired: 2 in, 2 out]
              }
            }
          }
        }
        n218 = property on="Progress" class="Clust (strict)"("Visible"=FALSE) -> ()  [unwired: 2 in, 2 out]
      }
      event "Test Name": Mouse Enter {
        # "Populate the ring with the list of tests"
        n219 = event-data() -> ()  [unwired: 1 in, 1 out]
        n220 = call <vilib>:"NT Read String Array.vi"("Name"="/TestMode/TestList") -> ("String Array"=w354:string[])  [unwired: 9 in, 1 out]
        n221 = Build Array (concatenate)("Select the test to run...", w354) -> (w353:string[])
        n222 = property on="Test Name" class="Ring (strict)"("Strings []"=w353) -> ()  [unwired: 2 in, 2 out]
      }
      event "Test Name": Value Change {
        w356 = FALSE ("Visible")
        # "Tell the robot the test name to run"
        n223 = event-data() -> ("NewVal"=w360:u16)  [unwired: 1 in]
        n224 = property on="Test Name" class="Ring (strict)"() -> ("Strings []"=w361:string[])  [unwired: 2 in, 2 out]
        n225 = local write "Progress"(T6 {"Test Progress"=0, "Test Progress Text"=""} ("Progress")) -> ()
        n226 = Index Array(array=w361, index=w360) -> (element=w359:string)
        n227 = call <vilib>:"NT Write String.vi"("String"=w359, "Name"="/TestMode/TestName") -> ()  [unwired: 9 in, 1 out]
        n228 = property on="Progress" class="Clust (strict)"("Visible"=TRUE) -> ()  [unwired: 2 in, 2 out]
        n229 = property on="Motor" class="Clust (strict)"("Visible"=w356) -> ()  [unwired: 2 in, 2 out]
        n230 = property on="Test Slider" class="Slide (strict)"("Visible"=w356) -> ()  [unwired: 2 in, 2 out]
        n231 = property on="On/Off" class="Bool (strict)"("Visible"=w356) -> ()  [unwired: 2 in, 2 out]
        n232 = property on="Rev/Fwd" class="Clust (strict)"("Visible"=w356) -> ()  [unwired: 2 in, 2 out]
        n233 = property on="Test Ring" class="Ring (strict)"("Visible"=w356) -> ()  [unwired: 2 in, 2 out]
      }
      event "Auto List": Mouse Enter {
        # "Populate the combo box with the list of autonomous options"
        n234 = event-data() -> ()  [unwired: 1 in, 1 out]
        n235 = call <vilib>:"NT Read String Array.vi"("Name"="Auto List") -> ("String Array"=w363:string[])  [unwired: 9 in, 1 out]
        n236 = property on="Auto List" class="CmbBox"("Strings[]"=w363) -> ()  [unwired: 2 in, 2 out]
      }
      event "Auto List": Value Change {
        # "User modified the Auto Selection. Write to NT variable so robot knows."
        n237 = event-data() -> ("NewVal"=w366:string)  [unwired: 1 in]
        n238 = call <vilib>:"NT Write String.vi"("String"=w366, "Name"="Auto Selector") -> ()  [unwired: 9 in, 1 out]
      }
      event "Command Selection": Value Change {
        # "Get the params and show in table"
        n239 = event-data() -> ("NewVal"=w372:i32)  [unwired: 1 in]
        n240 = property on="Command Selection" class="MCListbox (strict)"() -> ("ItemNames"=w370:string[][])  [unwired: 2 in, 2 out]
        n241 = call <vilib>:"WPI_DashboardUpdate Command Params.vi"("NewVal"=w372, "Commands"=w370, "Param Tbl"=w371) -> ()  [unwired: 8 in, 1 out]
      }
      event "Execute Command": Value Change {
        # "Started one, Unique ID holds\nresponse"
        n242 = event-data() -> ()  [unwired: 1 in, 1 out]
        n243 = property on="Command Selection" class="MCListbox (strict)"() -> ("ItemNames"=w383:string[][])  [unwired: 2 in, 2 out]
        n244 = Index Array(array=w383, index (row)="Command Selection", index (col)=0) -> (element=w381:string)
        n245 = call <vilib>:"Invoke Commands.vi"("Command Params"="Command Params", "Function Name"=w381) -> ("Params"=w377:u8, "Started"=w376:bool)  [unwired: 7 in, 1 out]
        n246 = Array Subset(array="Command Params", length (row)=w377) -> (w378:string[][])  [unwired: 3 in]
        n247 = Select(t="Executing" ("Cmd Status"), s=w376, f="" ("Cmd Status")) -> (s? t:f=→"Cmd Status":string)
      }
      event "Command Selection": Double Click {
        n248 = event-data() -> ("Row"=w391:i32)  [unwired: 1 in]
        n249 = property on="Command Selection" class="MCListbox (strict)"() -> ("ItemNames"=w394:string[][])  [unwired: 2 in, 2 out]
        n250 = local read "Command Params"() -> (w390:string[][])
        n251 = Index Array(array=w394, index (row)=w391, index (col)=0) -> (element=w392:string)
        n252 = call <vilib>:"Invoke Commands.vi"("Command Params"=w390, "Function Name"=w392) -> ("Params"=w389:u8, "Started"=w384:bool)  [unwired: 7 in, 1 out]
        n253 = Array Subset(array=w390, length (row)=w389) -> (w388:string[][])  [unwired: 3 in]
        n254 = Select(t="Executing" ("Cmd Status"), s=w384, f="" ("Cmd Status")) -> (s? t:f=w385:string)
        n255 = local write "Cmd Status"(w385) -> ()
      }
      event "CheckList": Double Click {
        # "Shift clears all"
        # "Update symbols on the listbox"
        n256 = event-data() -> ("PlatMods.Shift"=w396:bool, "Row"=w398:i32)  [unwired: 1 in]
        n257 = case shown="True" w396 {
          tunnel: w398 -> [w402 _]
          tunnel: 1 -> [w401 _]
          frame False {
            n258 = property on="CheckList" class="LstBox (strict)"() -> ("Item Symbols"=w400:i32[])  [unwired: 2 in, 2 out]
            n259 = Replace Array Subset(array=w400, new element=w401, index=w402) -> (w399:i32[])
            n260 = property on="CheckList" class="LstBox (strict)"("Item Symbols"=w399) -> ()  [unwired: 2 in, 2 out]
          }
          frame True {
            w403 = 0 ("Top Row")
            n261 = property on="CheckList" class="LstBox (strict)"() -> ("Number of Rows"=w405:u32)  [unwired: 2 in, 2 out]
            n262 = Initialize Array(0, w405) -> (w404:i32[])
            n263 = property on="CheckList" class="LstBox (strict)"("Top Row"=w403, "Value"=w403, "Item Symbols"=w404) -> ()  [unwired: 2 in, 2 out]
          }
        }
      }
      event "CheckList": Key Down {
        # "Update symbols on the listbox\nLeft and right keys check and uncheck"
        n264 = event-data() -> ("VKey"=w409:T19)  [unwired: 1 in]
        n265 = case shown="\"Left\", \"Right\"" w409 {
          selector: w409 -> [w414 _]
          tunnel: eventvkey."Left" ("VKey") -> [w412 _]
          frame "Left", "Right" {
            n266 = Equal?(x=w412, y=w414) -> (x = y?=w413:bool)
            n267 = Select(t=0, s=w413, f=1) -> (s? t:f=w415:i32)
            n268 = property on="CheckList" class="LstBox (strict)"() -> ("Item Symbols"=w418:i32[])  [unwired: 2 in, 2 out]
            n269 = Replace Array Subset(array=w418, new element=w415, index="CheckList") -> (w417:i32[])
            n270 = property on="CheckList" class="LstBox (strict)"("Item Symbols"=w417) -> ()  [unwired: 2 in, 2 out]
          }
          frame Default {
          }
        }
      }
      event "Motor.Enable": Value Change {
        # "When the test mode otor enable helper is set, update that\ntree row item's value"
        n271 = event-data() -> ("NewVal"=w424:bool)  [unwired: 1 in]
        n272 = Unbundle("Motor") -> ("Value"=w423:dbl)  [unwired: 1 out]
        n273 = Select(t=w423, s=w424, f=0.0) -> (s? t:f=w421:dbl)
        n274 = call <vilib>:"NT Write Number.vi"("Numeric"=w421, "Name"=w420) -> ()  [unwired: 9 in, 1 out]
      }
      event "Test Slider": Value Change {
        # "When the test mode slider helper is set, update that\ntree row item's value"
        n275 = event-data() -> ("NewVal"=w427:dbl)  [unwired: 1 in]
        n276 = call <vilib>:"NT Write Number.vi"("Numeric"=w427, "Name"=w428) -> ()  [unwired: 9 in, 1 out]
      }
      event "On/Off": Value Change {
        # "When the test mode on/off helper value is set, update that\ntree row item's value"
        n277 = event-data() -> ("NewVal"=w432:bool)  [unwired: 1 in]
        n278 = Boolean To (0,1)(Boolean=w432) -> (0, 1=w431:i16)
        n279 = call <vilib>:"NT Write Number.vi"("Numeric"=w431, "Name"=w430) -> ()  [unwired: 9 in, 1 out]
      }
      event "Rev/Fwd": Value Change {
        # "When the test mode helper value for relays is set, update that\ntree row item's value"
        n280 = event-data() -> ("NewVal.Forward"=w440:bool, "NewVal.Reverse"=w439:bool)  [unwired: 1 in]
        n281 = Boolean To (0,1)(Boolean=w440) -> (0, 1=w436:i16)
        n282 = Boolean To (0,1)(Boolean=w439) -> (0, 1=w438:i16)
        n283 = Negate(x=w438) -> (-x=w437:i16)
        n284 = Add(x=w436, y=w437) -> (x+y=w435:i16)
        n285 = call <vilib>:"NT Write Number.vi"("Numeric"=w435, "Name"=w434) -> ()  [unwired: 9 in, 1 out]
      }
      event "Test Ring": Value Change {
        # "When a test mode helper value is selected from the ring,\nset the tree item's variable to the string value"
        n286 = event-data() -> ("NewVal"=w444:u16)  [unwired: 1 in]
        n287 = property on="Test Ring" class="Ring (strict)"() -> ("Strings []"=w445:string[])  [unwired: 2 in, 2 out]
        n288 = Index Array(array=w445, index=w444) -> (element=w443:string)
        n289 = call <vilib>:"NT Write String.vi"("String"=w443, "Name"=w442) -> ()  [unwired: 9 in, 1 out]
      }
      event "Rec Mode": Value Change {
        # "Update globals for recording mode and path to read log from.\nClear when logging and let NetworkTables set path for vision to\nuse."
        n290 = event-data() -> ("NewVal"=w456:enum32{"Stop", "Record", "Playback"})  [unwired: 1 in]
        n291 = global write "WPI_DashboardLogging Global.vi" "Logging Filename"(path "") -> ()
        n292 = global write "WPI_DashboardLogging Global.vi" "Recording"(w456) -> ()
        n293 = case shown="\"Playback\"" w456 {
          tunnel: w455 -> [_ w458 w467]
          tunnel: [_ _ w466] -> w453
          tunnel: [_ _ w465] -> _
          tunnel: w451 -> [_ _ w463]
          tunnel: cluster{i32, i32} {-250, 170} -> [_ _ w462]
          tunnel: [_ _ T20 {"Image Size"=TRUE, "Image Type"=TRUE, "Pixel Value"=TRUE, "ROI Information"=TRUE, "Zoom Factor"=FALSE} ("Image Information Shown:All Elements")] -> w449
          tunnel: [_ _ TRUE ("Zoom Factor")] -> w448
          tunnel: w447 -> [_ _ w459]
          frame Default {
          }
          frame "Stop", "Record" {
            # "Place Window too"
            n294 = invoke class="VI" method="FP.Close"(reference=w458) -> (reference out=w457:refnum<vi>)  [unwired: 2 in, 2 out]
            n295 = invoke class="VI" method="Abort VI"(reference=w457) -> ()  [unwired: 2 in, 3 out]
          }
          frame "Playback" {
            n296 = call "Open Playback Panel.vi"("Offset"=w462, "DB VI Ref"=w463, "Playback in"=w467) -> ("Playback out"=w464:refnum<vi>)  [unwired: 8 in]
            n297 = register-events(w464, w459) -> (reference out=w466:refnum<event-registration>, error out=w465:errorcluster)  [unwired: 2 in]
          }
        }
        n298 = property on="Camera Image" class="ImageControl"("Image Information Shown"=w449, "Image Information Visible"=w448) -> ()  [unwired: 2 in, 2 out]
        n299 = call <vilib>:"WPI_DashboardNT Log FieldName Cache.vi"("Operation"=enum16{"Lookup/Add", "Index", "Clear"}."Clear") -> ()  [unwired: 8 in, 3 out]
      }
      event Panel Close {
        w469 = enum32{"Stop", "Record", "Playback"}."Stop" ("Rec Mode")
        # "Playback window has been closed, abort"
        n300 = event-data() -> ()  [unwired: 1 in, 4 out]
        n301 = local write "Rec Mode"(w469) -> ()
        n302 = global write "WPI_DashboardLogging Global.vi" "Recording"(w469) -> ()
      }
      event Panel Close {
        # "Abort playback window and ourself"
        n303 = event-data() -> ()  [unwired: 1 in, 4 out]
        n304 = invoke class="VI" method="FP.Close"(reference=w473) -> (reference out=w472:refnum<vi>)  [unwired: 2 in, 2 out]
        n305 = invoke class="VI" method="Abort VI"(reference=w472) -> (error out=w471:errorcluster)  [unwired: 2 in, 2 out]
        n306 = invoke class="VI" method="Abort VI"(error in=w471) -> ()  [unwired: 2 in, 3 out]
      }
      event User Event {
        n307 = event-data() -> ("IDs"=w480:cluster{"RPC field ID":u16, "Unique ID":u16}, "String"=w479:string)  [unwired: 1 in]
        n308 = Bundle("IDs"=w480, "String"=w479) -> (w478:T8)  [unwired: 1 in]
        n309 = call <vilib>:"Retrieve RPC Response.vi"("RPC Response"=w478) -> ("Output"=w476:string[][])  [unwired: 10 in]
        n310 = Build Array (concatenate)(w474, w476) -> (w475:string[][])
        n311 = local write "Command Params"(w475) -> ()
        n312 = local write "Cmd Status"("" ("Cmd Status")) -> ()
      }
      event "Tree": Double Click {
        n313 = event-data() -> ("PlatMods"=w484:T23, "Tag"=w483:string)  [unwired: 1 in]
        n314 = Unbundle(w484) -> ("Shift"=w482:bool)  [unwired: 4 out]
        n315 = Not(x=w482) -> (.not. x?=w481:bool)
        n316 = call <vilib>:"NT Update Persistence.vi"("Persistence"=w481, "Name"=w483) -> ()  [unwired: 9 in, 1 out]
      }
    }
  }
  n317 = while {
    tunnel: w64 -> [w487]
    i -> [w490]
    stop <- FALSE stop-if-true
    n318 = Wait (ms)(milliseconds to wait=u32 100) -> ()  [unwired: 1 out]
    n319 = case shown="\"Playback\"" "Rec Mode" {
      tunnel: w490 -> [_ _ w505]
      tunnel: [u32 2829099 ("Base Color") u32 11141120 ("Target Color") w494] -> w486
      frame "Stop", Default {
        # "Reset the color, extra updates don't cost much"
      }
      frame "Record" {
      }
      frame "Playback" {
        # "Playback"
        n320 = Quotient & Remainder(x=w505, y=u32 50 ("milliseconds to wait")) -> (x-y*floor(x/y)=w501:u32)  [unwired: 1 out]
        n321 = Divide(x=w501, y=u32 50 ("milliseconds to wait")) -> (x/y=w498:dbl)
        n322 = Multiply(x=6.283185307179586, y=w498) -> (x*y=w503:dbl)
        n323 = Sine(x=w503) -> (sin(x)=w502:dbl)
        n324 = Absolute Value(x=w502) -> (abs(x)=w495:dbl)
        n325 = call "Interpolate RGB Color.vi"("Proportion"=w495, "Target Color"=u32 30976, "Base Color"=u32 2829099) -> ("Result Color"=w494:u32)  [unwired: 8 in]
      }
    }
    n326 = property class="Pane"(reference=w487, "PaneColor"=w486) -> ()  [unwired: 1 in, 2 out]
  }
  n327 = local write "Dashboard Tab"(T2."Drive" ("Dashboard Tab")) -> ()
  n328 = property on="On/Off" class="Bool (strict)"("Visible"=w33) -> ()  [unwired: 2 in, 2 out]
  n329 = property on="Motor" class="Clust (strict)"("Visible"=w33) -> ()  [unwired: 2 in, 2 out]
  n330 = property on="Progress" class="Clust (strict)"("Visible"=w33) -> ()  [unwired: 2 in, 2 out]
  n331 = property on="Test Ring" class="Ring (strict)"("Visible"=w33) -> ()  [unwired: 2 in, 2 out]
  n332 = property on="Rev/Fwd" class="Clust (strict)"("Visible"=w33) -> ()  [unwired: 2 in, 2 out]
  n333 = while {
    tunnel: u16 1741 ("timeout ms (25000)") -> [w507]
    stop <- FALSE stop-if-true
    n334 = TCP Create Listener(10:w507) -> (0:w506:errorcluster, 3:w508:refnum<k5>)  [unwired: 4 in, 1 out]
    n335 = case shown="No Error" w506 {
      selector: w506 -> [w510 _]
      tunnel: w508 -> [w511 _]
      frame No Error {
        n336 = while {
          tunnel: w511 -> [w514]
          tunnel: w510 -> [w513]
          stop <- FALSE stop-if-true
          n337 = TCP Wait On Listener(8:w513, 11:w514) -> (0:w515:errorcluster, 4:w516:refnum<k5>)  [unwired: 2 in, 3 out]
          n338 = local write "TCP"(w516) -> ()
          n339 = case shown="No Error" w515 {
            frame No Error {
            }
            frame Error {
              n340 = Wait (ms)(milliseconds to wait=u32 1000) -> ()  [unwired: 1 out]
            }
          }
        }
      }
      frame Error {
        n341 = Wait (ms)(milliseconds to wait=u32 1000) -> ()  [unwired: 1 out]
      }
    }
  }
  n342 = local write "Command Selection"(u16 0 ("milliseconds to wait")) -> ()
  n343 = local write "Command Params"(string[][] [] ("Command Params")) -> ()
  n344 = global write "WPI_DashboardLogging Global.vi" "Recording"(w58) -> ()
  n345 = local write "Rec Mode"(w58) -> ()
  n346 = call <vilib>:"NT Write String.vi"("String"="Auto List", "Name"="Auto List") -> ()  [unwired: 9 in, 1 out]
